vi "Stop Core.vi"(10 "final error code":i32, 11 "Configuration in":refnum<class "Configuration.lvclass">) -> (3 "Configuration out":refnum<class "Configuration.lvclass">)   [LabVIEW 2017, in "Configuration.lvlib" / "Configuration.lvclass"]
doc: "(<B>Filename</B>: Actor Framework.lvlib:Actor.lvclass:Stop Core.vi)\n\nDefines what the actor does before it stops. Use the <B>final error code</B> input to determine whether the actor shut down in response to an error.\n\nBy default, this method does nothing. A descendant class may override it to define behavior, such as shutting down any processes the actor initiated in its override of the Actor Core method."
uses:
  Configuration.lvclass
  Configuration.lvclass/Configuration.ctl
  <vilib>/ActorFramework/Actor/Actor.lvclass
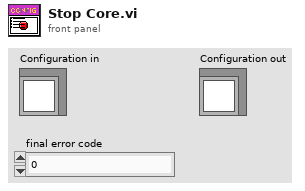
[diagram p1: front panel]
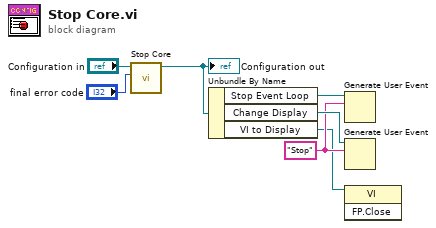
[diagram p0: block diagram]
diagram:
  w2 = "Stop" ("event data")
  n1 = call-parent "Stop Core.vi"("final error code"="final error code", "Actor in"="Configuration in") -> ("Actor out"=w5:refnum<class "Configuration.lvclass">)  [unwired: 9 in]
  "Configuration out" <- w5
  n2 = Unbundle By Name(w5) -> ("Stop Event Loop"=w3:refnum<user-event>, "Change Display"=w4:refnum<user-event>, "VI to Display"=w1:refnum<vi>)
  n3 = Generate User Event(user event=w3, event data cluster=w2) -> ()  [unwired: 2 in, 2 out]
  n4 = Generate User Event(user event=w4, event data cluster=w2) -> ()  [unwired: 2 in, 2 out]
  n5 = invoke class="VI" method="FP.Close"(reference=w1) -> ()  [unwired: 2 in, 3 out]
